vi "Write Dirty.vi"(8 "error in (no error)":errorcluster, 10 "Dirty":bool, 11 "CellDirtyStateChanged in":refnum<class "CellDirtyStateChanged.lvclass">) -> (0 "error out":errorcluster, 3 "CellDirtyStateChanged out":refnum<class "CellDirtyStateChanged.lvclass">)   [LabVIEW 2013, in "DataGrid.lvlib" / "CellDirtyStateChanged.lvclass"]
uses:
  CellDirtyStateChanged.lvclass
  CellDirtyStateChanged.lvclass/CellDirtyStateChanged.ctl
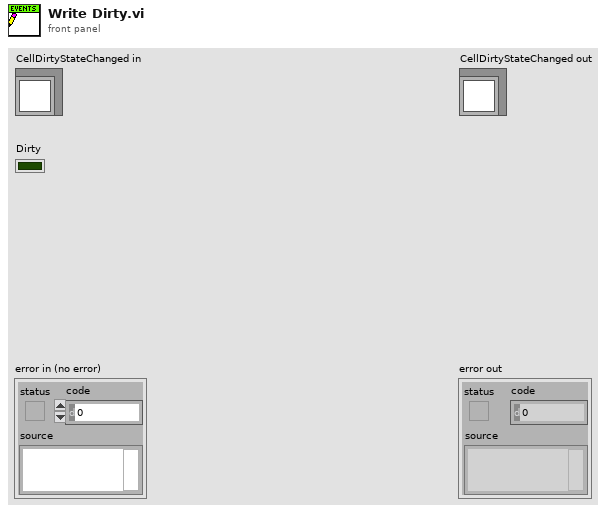
[diagram p1: front panel]
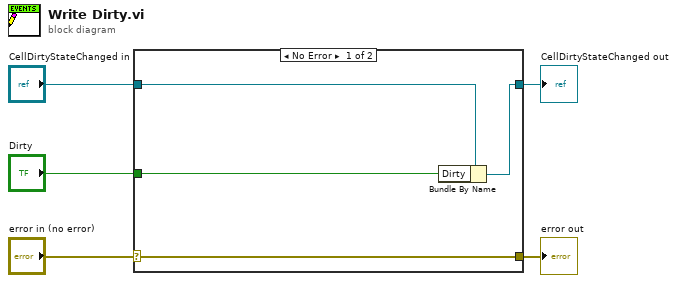
[diagram p0: block diagram]
diagram:
  n1 = case shown="No Error" "error in (no error)" {
    selector: "error in (no error)" -> [w9 w10]
    tunnel: [w9 w10] -> w4
    tunnel: [w7 w11] -> w2
    tunnel: "CellDirtyStateChanged in" -> [w8 w11]
    tunnel: "Dirty" -> [w6 _]
    frame No Error {
      n2 = Bundle By Name(cluster=w8, "Dirty"=w6) -> (w7:refnum<class "CellDirtyStateChanged.lvclass">)
    }
    frame Error {
    }
  }
  "error out" <- w4
  "CellDirtyStateChanged out" <- w2
